vi "Get Switch Heater State.vi"(3 "error in":T1, 5 "VISA resource name":refnum<visa-resource-name>) -> (0 "error out":T1, 1 "Switch Heater state":bool, 2 "VISA resource name out":refnum<visa-resource-name>)   [LabVIEW 2019]
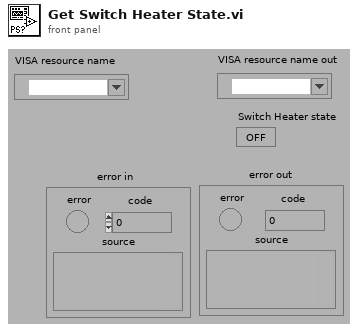
[diagram p1: front panel]
types:
  T1 = cluster{"error":bool, "code":i32, "source":string}
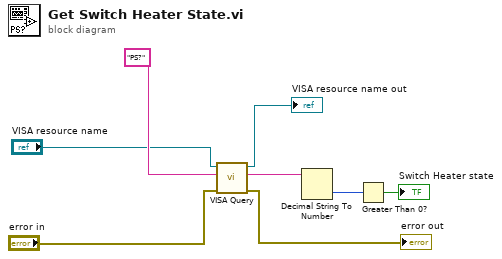
[diagram p0: block diagram]
diagram:
  n1 = call "VISA Query.vi"("error in (no error)"="error in", "Command"="PS?", "VISA resource name"="VISA resource name") -> ("error out"=→"error out":errorcluster, "Response"=w4:string, "VISA resource name out"=→"VISA resource name out":refnum<visa-resource-name>)  [unwired: 4 in, 2 out]
  n2 = Decimal String To Number(string=w4) -> (number=w8:i32)  [unwired: 2 in, 1 out]
  n3 = Greater Than 0?(x=w8) -> (x > 0?=→"Switch Heater state":bool)
